vi "Read Step Name.vi"(8 "error in (no error)":errorcluster, 11 "Result in":refnum<class "Result.lvclass">) -> (0 "error out":errorcluster, 2 "Step Name":string, 3 "Result out":refnum<class "Result.lvclass">)   [LabVIEW 2015, in "Result.lvclass"]
uses:
  Result.lvclass
  Result.lvclass/Result.ctl
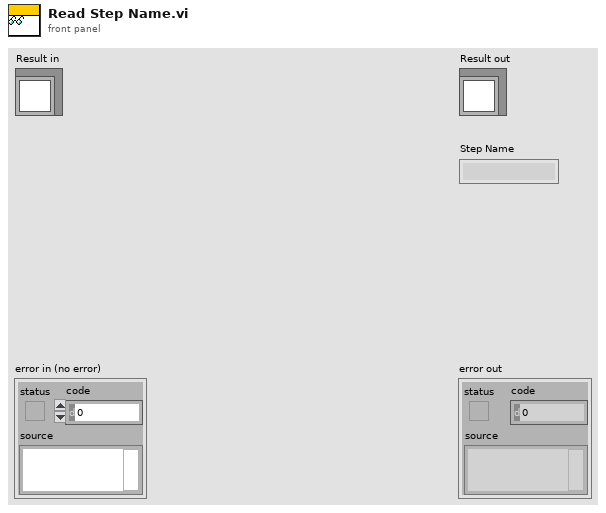
[diagram p1: front panel]
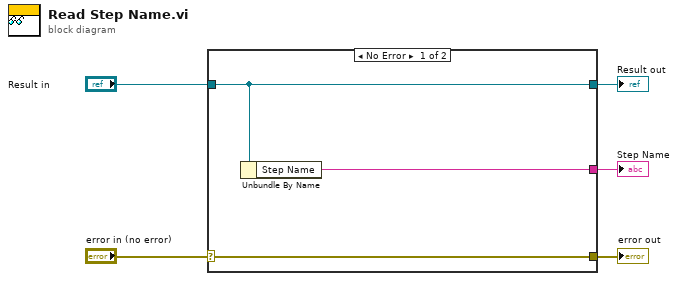
[diagram p0: block diagram]
diagram:
  n1 = case shown="No Error" "error in (no error)" {
    selector: "error in (no error)" -> [w8 w9]
    tunnel: [w8 w9] -> w4
    tunnel: [w7 w10] -> w2
    tunnel: "Result in" -> [w7 w10]
    tunnel: [w6 _] -> w1
    frame No Error {
      n2 = Unbundle By Name(w7) -> ("Step Name"=w6:string)
    }
    frame Error {
    }
  }
  "error out" <- w4
  "Result out" <- w2
  "Step Name" <- w1
